vi "Read.vi"(7 "timeout in ms (-1)":i32=-1, 10 "channel":T1) -> (1 "last element?":bool, 2 "element":T2, 3 "element valid?":bool, 5 "timed out?":bool, 6 "count":i32)   [LabVIEW 2017, in "Stream-t'WPI_EncoderType.ctl'.lvlib"]
doc: "Reads an element from a Stream channel. The endpoint waits if the channel is empty."
uses:
  <extravilib>/ChannelInstances/Stream-t'WPI_EncoderType.ctl'.lvlib
  <vilib>/Rock Robotics/WPI/Encoder/WPI_EncoderType.ctl
  <extravilib>/ChannelInstances/Stream-t'WPI_EncoderType.ctl'/)Channel.ctl
  <resource>/ChannelSupport/_ChannelSupport/WaitIfNeeded.vi
  <extravilib>/ChannelInstances/Stream-t'WPI_EncoderType.ctl'/)Channel.vi
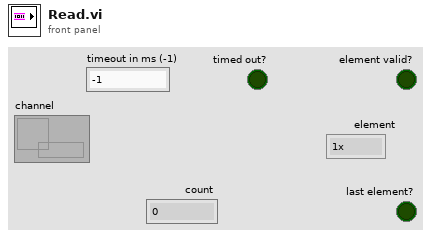
[diagram p1: front panel]
types:
  T1 = typedef "Stream-t'WPI_EncoderType.ctl'.lvlib/)Channel.ctl" = refnum<queue>
  T2 = typedef "WPI_EncoderType.ctl" = enum16{"1x", "2x", "4x"}
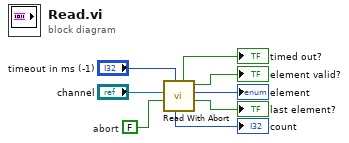
[diagram p0: block diagram]
diagram:
  w1 = FALSE  # abort
  n1 = call <extravilib>:"Read With Abort.vi"("timeout in ms (-1)"="timeout in ms (-1)", "abort"=w1, "channel"="channel") -> ("last element?"=→"last element?":bool, "element"=→"element":T2, "element valid?"=→"element valid?":bool, "timed out?"=→"timed out?":bool, "count"=→"count":i32)  [unwired: 3 in, 1 out]
